vi "InfoSERI.vi"(8 "ExitSendCmd":bool, 11 "base path":path) -> (0 "NewCase?":bool, 1 "FileName":string, 3 "Patient Info Out":T1={"Eye Selector"=enum."Right", "Plane"=1, "First Name"="", "Last Name"="", "Notes"="", "Patient ID"="", "Scan Location"=enum."Radio Selection 1"} {"Plane" min=1 max=12 step=1 scale=0.0..12.0})   [LabVIEW 2022 SP3]
uses:
  -RT_support/PatientInfoDef.ctl
  Patient Routines/PatientGlobals.vi
  ScanningControl/Motion Controllers/-MotionRoutines/MotionGlobals.vi
panel:
  in  "Patient Info":T1={"Eye Selector"=enum."Right", "Plane"=12, "First Name"="", "Last Name"="", "Notes"="", "Patient ID"="", "Scan Location"=enum."Radio Selection 1"} {"Plane" min=1 max=12 step=1 scale=0.0..12.0}
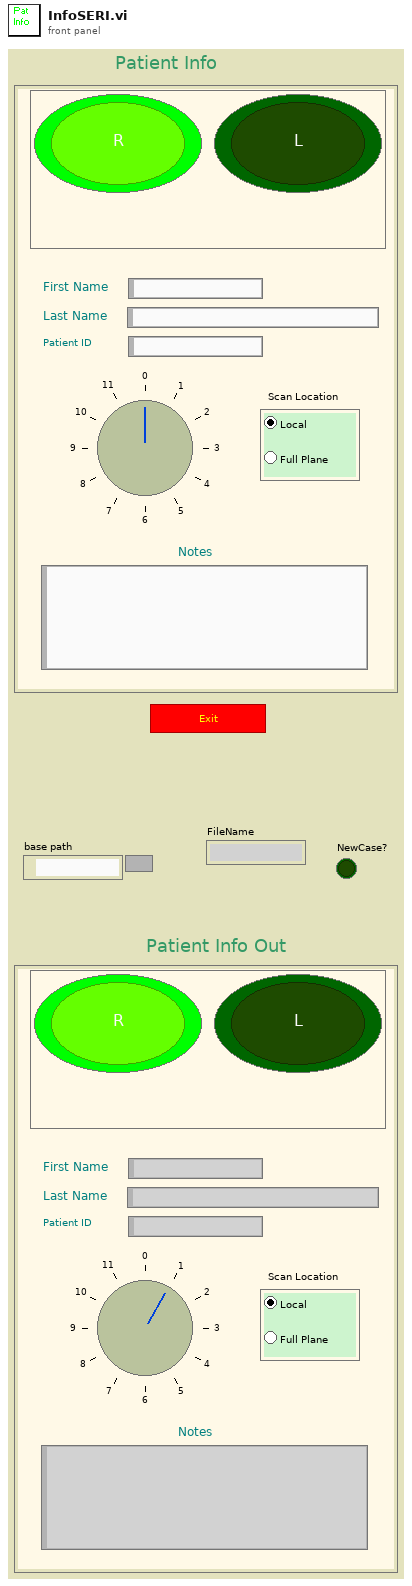
[diagram p1: front panel]
types:
  T1 = typedef "PatientInfoDef.ctl" = cluster{"Eye Selector":enum32{"Left", "Right"}, "Plane":i8, "First Name":string, "Last Name":string, "Notes":string, "Patient ID":string, "Scan Location":enum32{"Radio Selection 1", "Radio Selection 2"}}
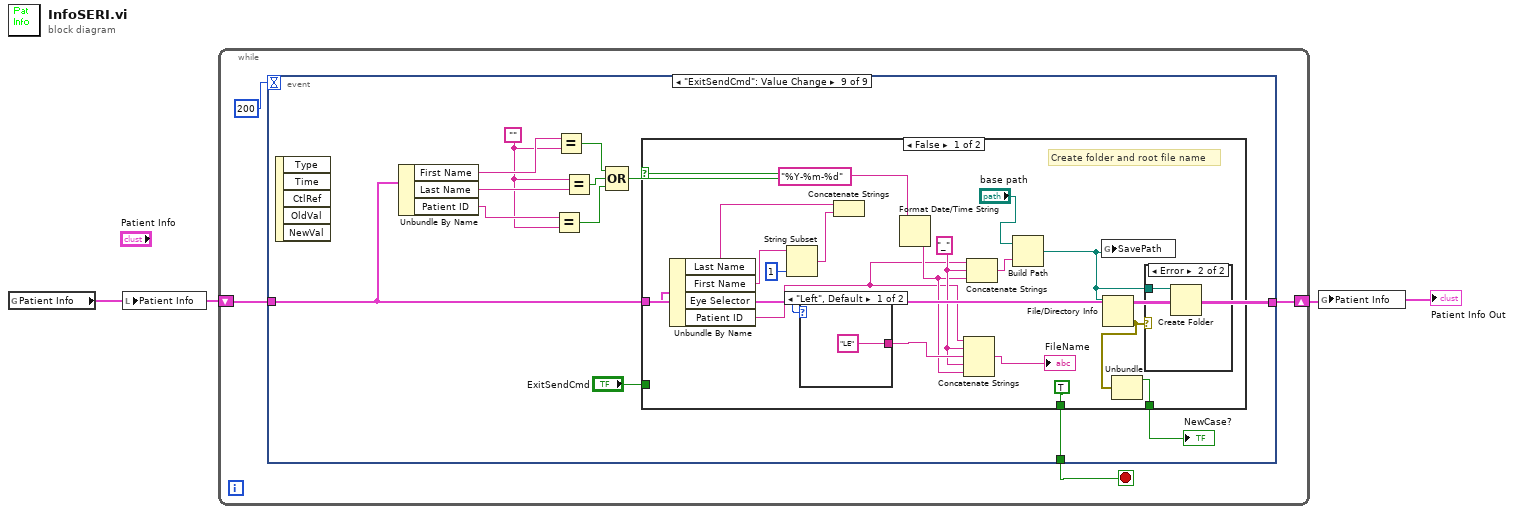
[diagram p0: block diagram]
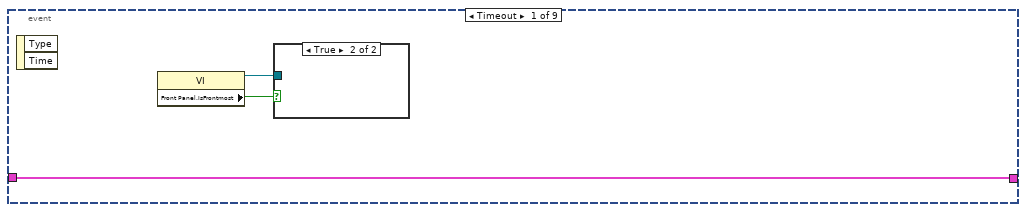
[diagram p2: hidden frame]
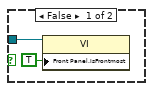
[diagram p3: hidden frame]
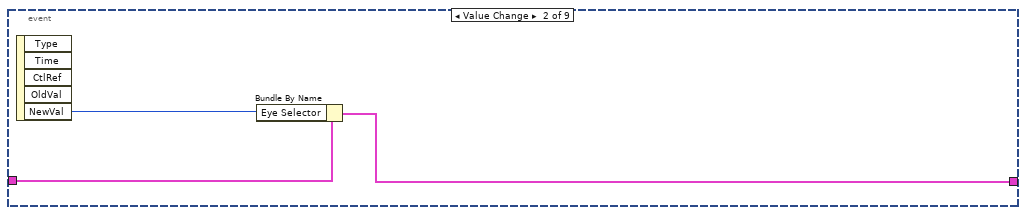
[diagram p4: hidden frame]
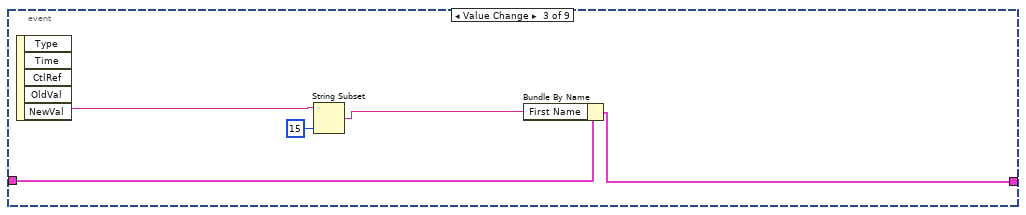
[diagram p5: hidden frame]
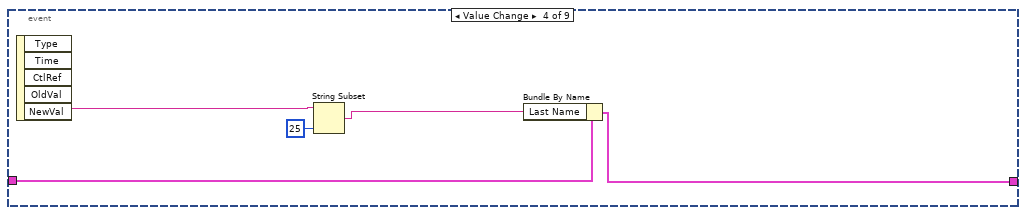
[diagram p6: hidden frame]
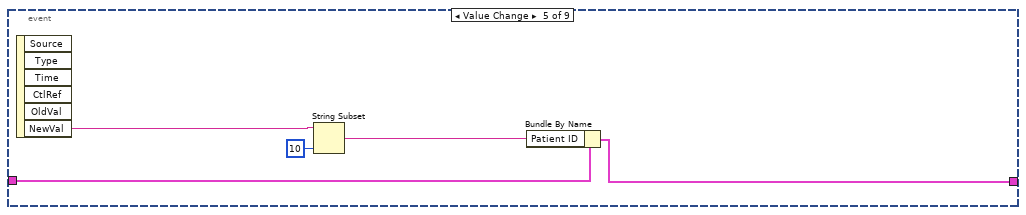
[diagram p7: hidden frame]
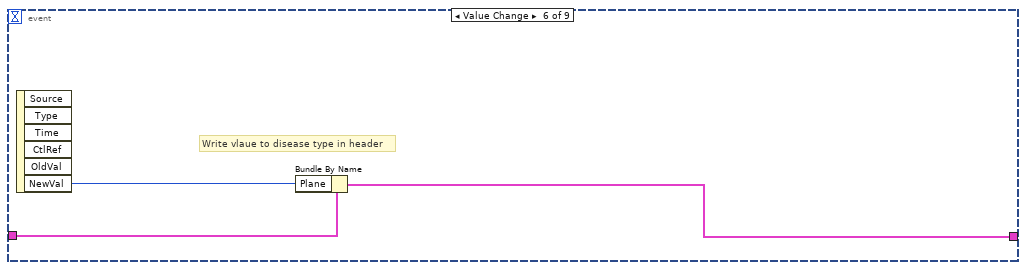
[diagram p8: hidden frame]
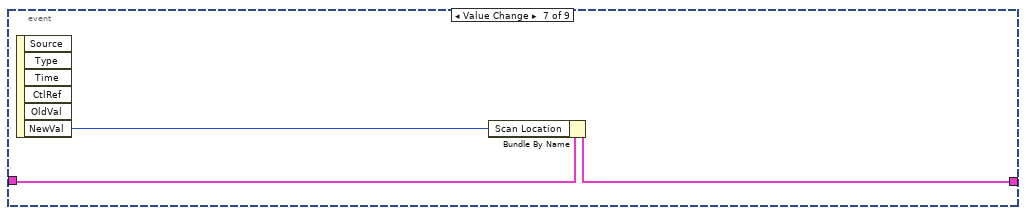
[diagram p9: hidden frame]
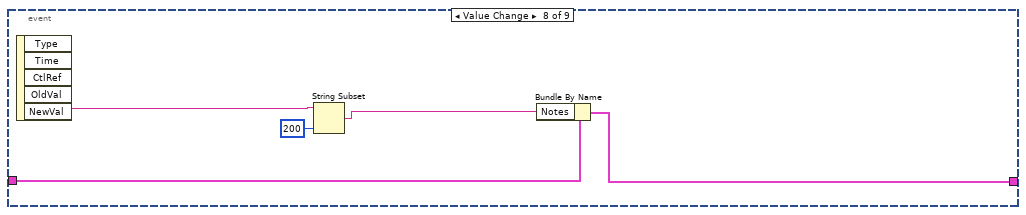
[diagram p10: hidden frame]
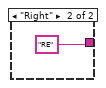
[diagram p12: hidden frame]
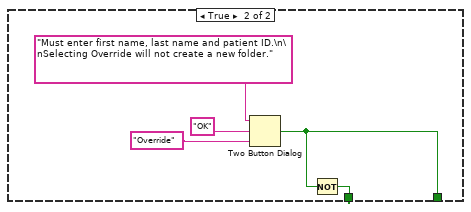
[diagram p13: hidden frame]
diagram:
  n1 = global read "PatientGlobals.vi" "Patient Info"() -> (w2:T1)
  n2 = local write "Patient Info"(w2) -> ()
  n3 = while {
    shift-right: [w6] -> w1
    shift-left: w2 -> [w5]
    stop <- w3 stop-if-true
    n4 = event shown="[8] \"ExitSendCmd\": Value Change" {
      selector: _ -> [_ _ _ _ _ _ _ _ _]
      dyn-events: _ -> [_ _ _ _ _ _ _ _ _]
      timeout: 200 -> [_ _ _ _ _ _ _ _ _]
      tunnel: [w9 w13 w15 w20 w26 w31 w34 w36 w42] -> w6
      tunnel: w5 -> [w9 w14 w16 w21 w27 w32 w35 w37 w42]
      tunnel: [_ _ _ _ _ _ _ _ w48] -> w3
      event Timeout {
        n5 = event-data() -> ()  [unwired: 1 in, 2 out]
        n6 = property class="VI"() -> (reference out=w7:refnum<vi>, "Front Panel.IsFrontmost"=w8:bool)  [unwired: 2 in, 1 out]
        n7 = case shown="True" w8 {
          tunnel: w7 -> [w10 _]
          frame False {
            n8 = property class="VI"(reference=w10, "Front Panel.IsFrontmost"=TRUE ("Front Panel Window:Is Frontmost")) -> ()  [unwired: 1 in, 2 out]
          }
          frame True {
          }
        }
      }
      event Value Change {
        n9 = event-data() -> ("NewVal"=w12:enum32{"Left", "Right"})  [unwired: 1 in, 4 out]
        n10 = Bundle By Name(cluster=w14, "Eye Selector"=w12) -> (w13:T1)
      }
      event Value Change {
        n11 = event-data() -> ("NewVal"=w19:string)  [unwired: 1 in, 4 out]
        n12 = String Subset(string=w19, length (rest)=15 ("length (rest)")) -> (substring=w17:string)  [unwired: 1 in]
        n13 = Bundle By Name(cluster=w16, "First Name"=w17) -> (w15:T1)
      }
      event Value Change {
        n14 = event-data() -> ("NewVal"=w24:string)  [unwired: 1 in, 4 out]
        n15 = String Subset(string=w24, length (rest)=25 ("length (rest)")) -> (substring=w22:string)  [unwired: 1 in]
        n16 = Bundle By Name(cluster=w21, "Last Name"=w22) -> (w20:T1)
      }
      event Value Change {
        n17 = event-data() -> ("NewVal"=w25:string)  [unwired: 1 in, 5 out]
        n18 = String Subset(string=w25, length (rest)=10 ("length (rest)")) -> (substring=w28:string)  [unwired: 1 in]
        n19 = Bundle By Name(cluster=w27, "Patient ID"=w28) -> (w26:T1)
      }
      event Value Change {
        # "Write vlaue to disease type in header"
        n20 = event-data() -> ("NewVal"=w30:i8)  [unwired: 1 in, 5 out]
        n21 = Bundle By Name(cluster=w32, "Plane"=w30) -> (w31:T1)
      }
      event Value Change {
        n22 = event-data() -> ("NewVal"=w33:enum32{"Radio Selection 1", "Radio Selection 2"})  [unwired: 1 in, 5 out]
        n23 = Bundle By Name(cluster=w35, "Scan Location"=w33) -> (w34:T1)
      }
      event Value Change {
        n24 = event-data() -> ("NewVal"=w40:string)  [unwired: 1 in, 4 out]
        n25 = String Subset(string=w40, length (rest)=200 ("length (rest)")) -> (substring=w38:string)  [unwired: 1 in]
        n26 = Bundle By Name(cluster=w37, "Notes"=w38) -> (w36:T1)
      }
      event "ExitSendCmd": Value Change {
        w45 = ""
        n27 = event-data() -> ()  [unwired: 1 in, 5 out]
        n28 = Unbundle By Name(w42) -> ("First Name"=w52:string, "Last Name"=w47:string, "Patient ID"=w46:string)
        n29 = Equal?(x=w46, y=w45) -> (x = y?=w44:bool)
        n30 = Equal?(x=w52, y=w45) -> (x = y?=w51:bool)
        n31 = Equal?(x=w45, y=w47) -> (x = y?=w50:bool)
        n32 = Compound Arithmetic op=OR(w51, w50, w44) -> (w49:bool)
        n33 = case shown="False" w49 {
          tunnel: [TRUE ("ExitSendCmd") w75] -> w48
          tunnel: "ExitSendCmd" -> [_ _]
          tunnel: w42 -> [w69 _]
          tunnel: [w56 w74] -> w41
          frame False {
            w55 = "_"
            # "Create folder and root file name"
            n34 = Unbundle By Name(w69) -> ("Last Name"=w65:string, "First Name"=w67:string, "Eye Selector"=w68:enum32{"Left", "Right"}, "Patient ID"=w53:string)
            n35 = String Subset(string=w67, length (rest)=1 ("length (rest)")) -> (substring=w66:string)  [unwired: 1 in]
            n36 = case shown="\"Left\", Default" w68 {
              tunnel: ["LE" "RE"] -> w63
              frame "Left", Default {
              }
              frame "Right" {
              }
            }
            n37 = Concatenate Strings(w65, w66) -> ()  [unwired: 1 out]
            n38 = Format Date/Time String(time format string (%c)="%Y-%m-%d") -> (date/time string=w54:string)  [unwired: 2 in]
            n39 = Concatenate Strings(w53, w55, w63, w55, w54) -> (→"FileName":string)
            n40 = Concatenate Strings(w53, w55, w54) -> (w59:string)
            n41 = Build Path(base path="base path", name or relative path=w59) -> (appended path=w61:path)
            n42 = global write "MotionGlobals.vi" "SavePath"(w61) -> ()
            n43 = File/Directory Info(path=w61) -> (error out=w57:errorcluster)  [unwired: 1 in, 6 out]
            n44 = Unbundle(w57) -> ("status"=w56:bool)  [unwired: 2 out]
            n45 = case shown="Error" w57 {
              tunnel: w61 -> [_ w71]
              frame No Error {
              }
              frame Error {
                n46 = Create Folder(path (use dialog)=w71) -> ()  [unwired: 2 in, 3 out]
              }
            }
          }
          frame True {
            n47 = Two Button Dialog(message="Must enter first name, last name and patient ID.\n\nSelecting Override will not create a new folder.", 1:"Override" ("T button name (\"OK\")"), 2:"OK" ("F button name (\"Cancel\")")) -> (T button?=w74:bool)
            n48 = Not(x=w74) -> (.not. x?=w75:bool)
          }
        }
        "NewCase?" <- w41
      }
    }
  }
  "Patient Info Out" <- w1
  n49 = global write "PatientGlobals.vi" "Patient Info"(w1) -> ()
